vi "NT Update Persistence.vi"(8 "error in":errorcluster, 10 "Persistence":bool=TRUE, 11 "Name":string="Numeric") -> (0 "error out":errorcluster)   [LabVIEW 2025]
doc: "Update the persistence setting for the topic. This determines whether the value is stored to a file and loaded into memory during startup."
uses:
  ntcoreffi.dll
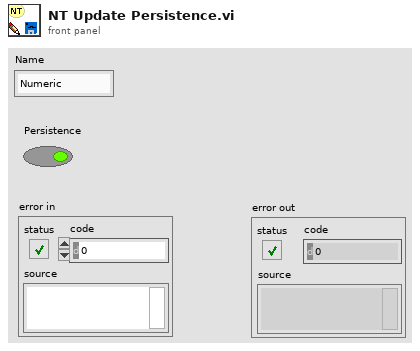
[diagram p1: front panel]
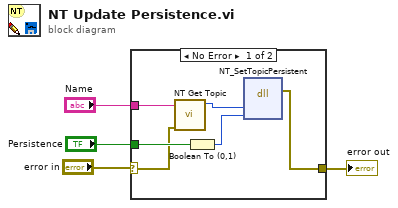
[diagram p0: block diagram]
diagram:
  n1 = case shown="No Error" "error in" {
    selector: "error in" -> [w6 w11]
    tunnel: "Persistence" -> [w8 _]
    tunnel: "Name" -> [w10 _]
    tunnel: [w5 w11] -> w2
    frame No Error {
      n2 = call <vilib>:"NT Get Topic.vi"("error in (no error)"=w6, "name"=w10) -> ("topicHandle"=w9:u32)  [unwired: 8 in, 1 out]
      n3 = Boolean To (0,1)(Boolean=w8) -> (0, 1=w7:i16)
      n4 = dll-call lib="ntcoreffi.*" fn="NT_SetTopicPersistent"("topicHandle"=w9, "value"=w7) -> (error out=w5:errorcluster)  [unwired: 6 in, 1 out]
    }
    frame Error {
    }
  }
  "error out" <- w2
